vi "Read Panel Helper.vi"(8 "Error In":errorcluster, 11 "Panel Actor in":refnum<class "Panel Actor.lvclass">) -> (0 "Error Out":errorcluster, 2 "Panel Helper":refnum<class "Panel Helper.lvclass">)   [LabVIEW 2023, in "Panel Actor.lvlib" / "Panel Actor.lvclass"]
doc: "Reads the Panel Helper for this Panel Actor.\n\nThe Panel Helper is only valid after this actors Pre-Launch init has run. Calling this VI before this will throw an error.\n\n<B>Panel Actor In:</B> Panel Actor object.\n<B>Error In:</B> Describes error conditions that occurred before this VI ran.\n\n<B>Panel Helpert:</B> Panel Helper object.\n<B>Error Out:</B> Contains error information.\n----\nPlease see the following web address for additional documentation and tutorial information:\nhttp://www.mooregoodideas.com/mgi-panel-manager/\n\nAuthor: Derek Trepanier\n\nCopyright (c) 2018, Moore Good Ideas, Inc.\n\nAll rights reserved.\n\nRedistribution and use in source and binary forms, with or without modification, are permitted provided that the following conditions are met:\n\n * Redistributions of source code must retain the above copyright notice, this list of conditions and the following disclaimer.\n * Redistributions in binary form must reproduce the above copyright notice, this list of conditions and the following disclaimer in the documentation and/or other materials provided with the distribution.\n * Neither the name of Moore Good Ideas, Inc. nor the names of its contributors may be used to endorse or promote products derived from this software without specific prior written permission.\n\nTHIS SOFTWARE IS PROVIDED BY THE COPYRIGHT HOLDERS AND CONTRIBUTORS \"AS IS\" AND ANY EXPRESS OR IMPLIED WARRANTIES, INCLUDING, BUT NOT LIMITED TO, THE IMPLIED WARRANTIES OF MERCHANTABILITY AND FITNESS FOR A PARTICULAR PURPOSE ARE DISCLAIMED. IN NO EVENT SHALL THE COPYRIGHT OWNER OR CONTRIBUTORS BE LIABLE FOR ANY DIRECT, INDIRECT, INCIDENTAL, SPECIAL, EXEMPLARY, OR CONSEQUENTIAL DAMAGES (INCLUDING, BUT NOT LIMITED TO, PROCUREMENT OF SUBSTITUTE GOODS OR SERVICES; LOSS OF USE, DATA, OR PROFITS; OR BUSINESS INTERRUPTION) HOWEVER CAUSED AND ON ANY THEORY OF LIABILITY, WHETHER IN CONTRACT, STRICT LIABILITY, OR TORT (INCLUDING NEGLIGENCE OR OTHERWISE) ARISING IN ANY WAY OUT OF THE USE OF THIS SOFTWARE, EVEN IF ADVISED OF THE POSSIBILITY OF SUCH DAMAGE."
uses:
  Library/Panel Actor.lvclass
  Panel/Panel Helper/Panel Helper.lvclass
  Library/Panel Actor.lvclass/Panel Actor.ctl
  <vilib>/Utility/error.llb/Error Cluster From Error Code.vi
  <vilib>/ErrorRing/Error Ring.xnode
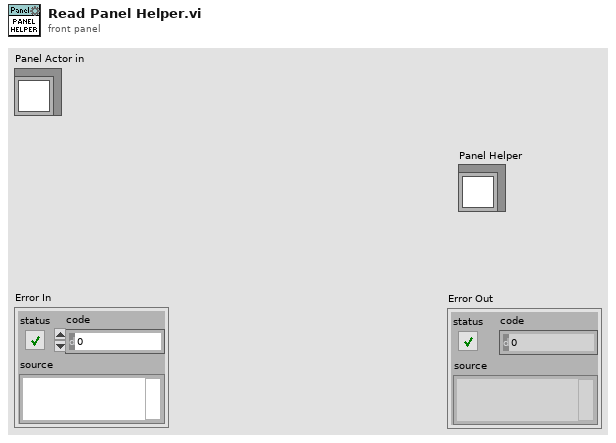
[diagram p1: front panel]
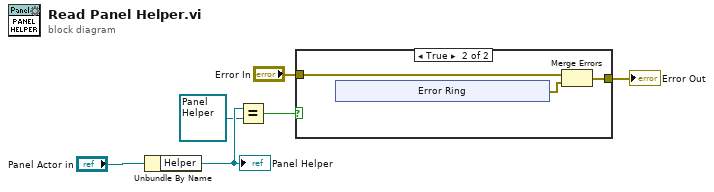
[diagram p0: block diagram]
diagram:
  n1 = Unbundle By Name("Panel Actor in") -> ("Helper"=w5:refnum<class "Panel Helper.lvclass">)
  "Panel Helper" <- w5
  n2 = Equal?(x=w5, y=refnum<class "Panel Helper.lvclass"> refnum) -> (x = y?=w1:bool)
  n3 = case shown="True" w1 {
    tunnel: "Error In" -> [w7 w10]
    tunnel: [w7 w9] -> w2
    frame False {
    }
    frame True {
      n4 = xnode "Error Ring"() -> ("error out"=w8:errorcluster)
      n5 = Merge Errors(w10, w8) -> (w9:errorcluster)
    }
  }
  "Error Out" <- w2
